vi "Find Controls in Data Dictionary.vi"(4 "output data dictionary":refnum<class "data dictionary.lvclass">, 6 "input data dictionary":refnum<class "data dictionary.lvclass">, 8 "error in (no error)":errorcluster, 10 "UI Refnum":refnum<vi>, 11 "channels in":refnum<class "TBM channel.lvclass">[](array[class])) -> (0 "error out":errorcluster, 2 "indicators":T1(array[cluster]), 3 "controls":T1(array[cluster]))   [LabVIEW 2014]
uses:
  <vilib>/NI/Tag Bus Module Framework/channel/TBM channel.lvclass
  <vilib>/NI/Tag Bus/dictionary/data dictionary.lvclass
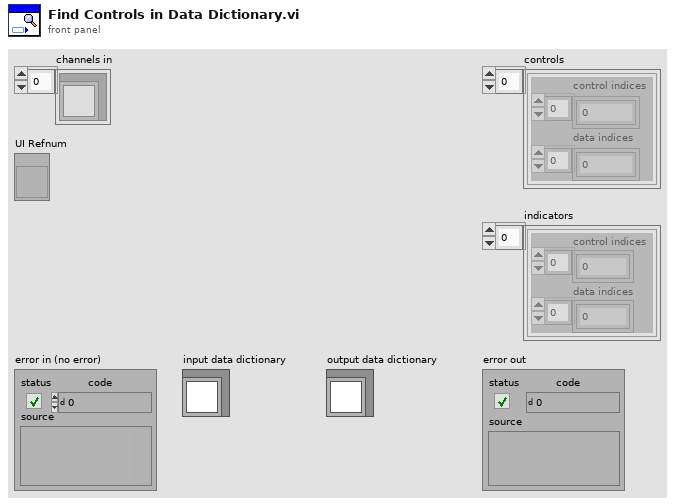
[diagram p1: front panel]
types:
  T1 = cluster{"control indices":i32[], "data indices":i32[]}[]
  T2 = typedef "TBM channel.lvclass/channel classification.ctl" = enum16{"input data", "output data", "processing parameter", "processing result"}
  T3 = typedef "tag bus.lvlib/tag descriptor.lvclass/Data Type.ctl" = enum16{"Double", "Single", "I64", "I32", "I16", "I8", "U64", "U32", "U16", "U8", "Boolean", "String", "Array of Double", "Array of Single", "Array of I64", "Array of I32", "Array of I16", "Array of I8", "Array of U64", "Array of U32", "Array of U16", "Array of U8", "Array of Boolean", "Array of String"}
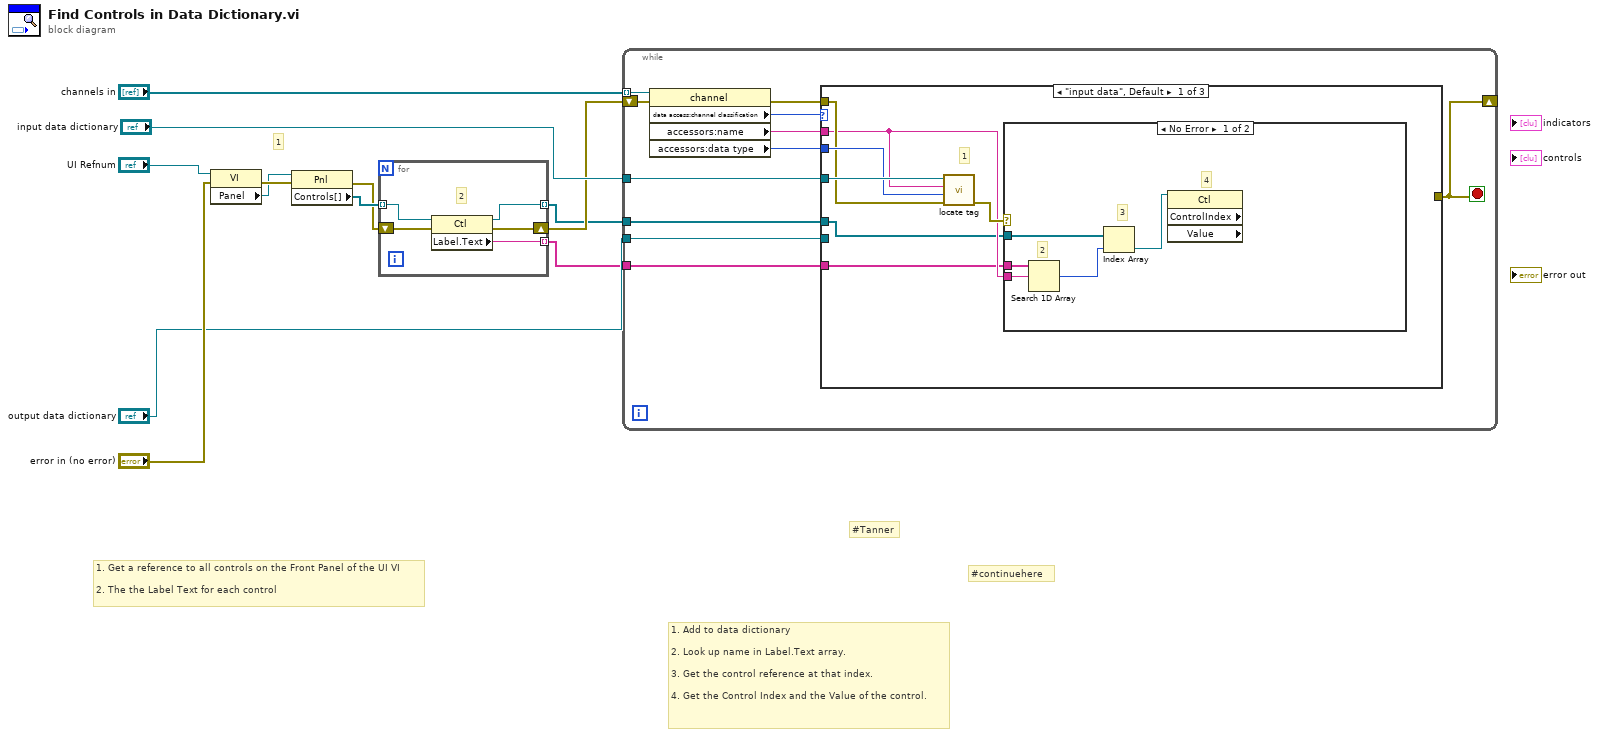
[diagram p0: block diagram]
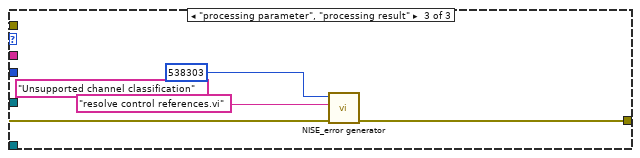
[diagram p4: hidden frame]
diagram:
  # "1. Add to data dictionary\n\n2. Look up name in Label.Text array.\n\n3. Get the control reference at that index.\n\n4. Get the Control Index and the Value of the control."
  # "#continuehere"
  # "#Tanner"
  # "1. Get a reference to all controls on the Front Panel of the UI VI\n\n2. The the Label Text for each control"
  # "1"
  n1 = property class="VI"(reference="UI Refnum", error in="error in (no error)") -> (error out=w10:errorcluster, "Panel"=w9:refnum<vi>)  [unwired: 1 out]
  n2 = property class="Pnl"(reference=w9, error in=w10) -> (error out=w7:errorcluster, "Controls[]"=w8:refnum<vi>[])  [unwired: 1 out]
  n3 = for {
    tunnel: w8 -> [w17] mode=indexing
    tunnel: [w16] -> w2 mode=indexing
    shift-right: [w15] -> w3
    shift-left: w7 -> [w14]
    tunnel: [w13] -> w1 mode=indexing
    # "2"
    n4 = property class="Ctl"(reference=w17, error in=w14) -> (reference out=w13:refnum<vi>, error out=w15:errorcluster, "Label.Text"=w16:string)
  }
  n5 = while {
    tunnel: "channels in" -> [w28] mode=indexing
    tunnel: "input data dictionary" -> [w23]
    tunnel: "output data dictionary" -> [w22]
    shift-right: [w20] -> _
    shift-left: w3 -> [w21]
    tunnel: w2 -> [w19]
    tunnel: w1 -> [w18]
    stop <- w20 stop-if-true
    n6 = property class="channel"(reference=w28, error in=w21) -> (error out=w26:errorcluster, "data access:channel classification"=w27:T2, "accessors:name"=w25:string, "accessors:data type"=w24:T3)  [unwired: 1 out]
    n7 = case shown="\"input data\", Default" w27 {
      tunnel: w26 -> [w33 _ w42]
      tunnel: [_ _ w41] -> w20
      tunnel: w25 -> [w31 _ _]
      tunnel: w24 -> [w34 _ _]
      tunnel: w23 -> [w35 _ _]
      tunnel: w22 -> [_ _ _]
      tunnel: w19 -> [w30 _ _]
      tunnel: w18 -> [w29 _ _]
      frame "input data", Default {
        # "1"
        n8 = call <vilib>:"locate tag.vi"("error in"=w33, "data type"=w34, "name"=w31, "data dictionary in"=w35) -> ("error out"=w32:errorcluster)  [unwired: 5 in, 2 out]
        n9 = case shown="No Error" w32 {
          tunnel: w31 -> [w40 _]
          tunnel: w30 -> [w39 _]
          tunnel: w29 -> [w37 _]
          frame No Error {
            # "4"
            # "3"
            # "2"
            n10 = Search 1D Array(1D array=w39, element=w40) -> (index of element=w38:i32)  [unwired: 1 in]
            n11 = Index Array(array=w37, index=w38) -> (element=w36:refnum<vi>)
            n12 = property class="Ctl" props=["ControlIndex", "Value"](reference=w36) -> ()  [unwired: 1 in, 4 out]
          }
          frame Error {
          }
        }
      }
      frame "output data" {
      }
      frame "processing parameter", "processing result" {
        n13 = call <vilib>:"NISE_error generator.vi"("error in"=w42, "source"="resolve control references.vi", "append error message"="Unsupported channel classification", "error code (0)"=538303) -> ("error out"=w41:errorcluster)  [unwired: 5 in]
      }
    }
  }
